vi "demo.vi"() -> ()   [LabVIEW 2016, in "mqtt.lvlib"]
uses:
  mqtt.lvlib
panel:
  in  "payload":string="Some message"
  in  "topicToPublish":string="test/device1"
  in  "topic":string="test/#"
  out "received":T1
  in  "sendSubscribe":bool
  in  "sendPublish":bool
  # "Subscribe"
  # "Subscribe"
  # "1. Connect to mqtt broker (server) by running mqtt.py\n2. Run this vi\n3. Subscribe to a topic\n4. Publish to the topic and it will be received by this vi\n5. Close panel to stop vi"
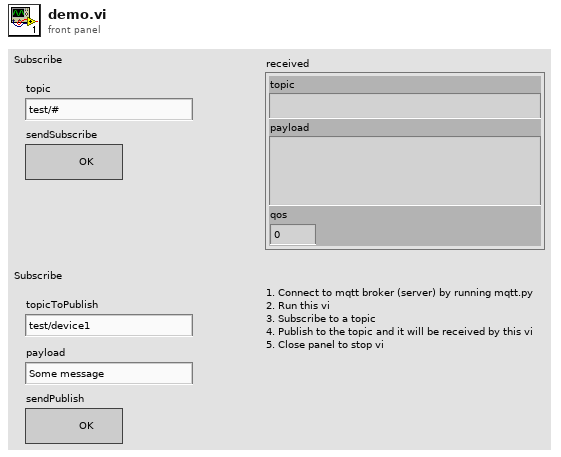
[diagram p1: front panel]
types:
  T1 = cluster{"topic":string, "payload":string, "qos":i32}
  T2 = enum16{"big-endian, network order", "native, host order", "little-endian"}
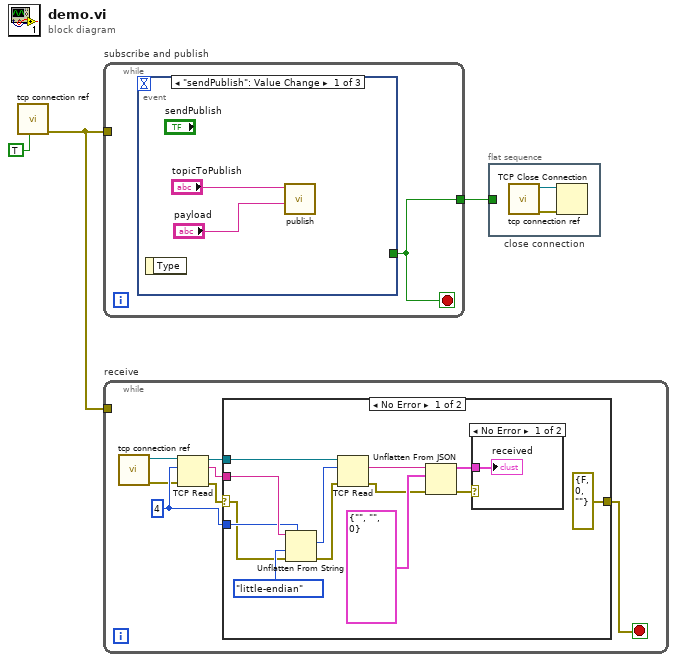
[diagram p0: block diagram]
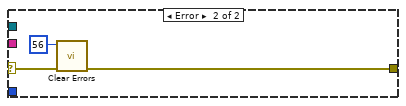
[diagram p3: hidden frame]
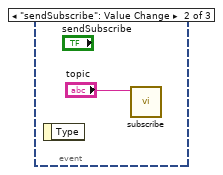
[diagram p4: hidden frame]
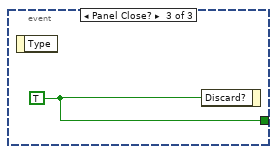
[diagram p5: hidden frame]
diagram:
  n1 = call "tcp connection ref.vi"("init"=TRUE) -> ("Error Out"=w2:errorcluster)  [unwired: 9 in, 1 out]
  n2 = while "subscribe and publish" {
    tunnel: w2 -> [_]
    tunnel: [w4] -> w1
    stop <- w4 stop-if-true
    n3 = event shown="[0] \"sendPublish\": Value Change" {
      selector: _ -> [_ _ _]
      dyn-events: _ -> [_ _ _]
      timeout: _ -> [_ _ _]
      tunnel: [_ _ w8] -> w4
      event "sendPublish": Value Change {
        n4 = event-data() -> ()  [unwired: 1 in, 1 out]
        n5 = call "publish.vi"("payload (something)"="payload", "topic (test/device1)"="topicToPublish") -> ()  [unwired: 9 in, 1 out]
      }
      event "sendSubscribe": Value Change {
        n6 = event-data() -> ()  [unwired: 1 in, 1 out]
        n7 = call "subscribe.vi"("topic (test/#)"="topic") -> ()  [unwired: 10 in, 1 out]
      }
      event Panel Close? {
        w8 = TRUE ("Discard?")
        n8 = event-data() -> ()  [unwired: 1 in, 1 out]
        n9 = event-data("Discard?"=w8) -> ()  [unwired: 1 in, 1 out]
      }
    }
  }
  n10 = while "receive" {
    tunnel: w2 -> [_]
    stop <- w9 stop-if-true
    w13 = 4 ("bytes to read")
    n11 = call "tcp connection ref.vi"() -> ("Error Out"=w11:errorcluster, "tcpRef"=w10:refnum<k5>)  [unwired: 10 in]
    n12 = TCP Read(connection ID=w10, bytes to read=w13, error in (no error)=w11) -> (connection ID out=w12:refnum<k5>, data out=w14:string, error out=w15:errorcluster)  [unwired: 2 in]
    n13 = case shown="No Error" w15 {
      selector: w15 -> [w19 w31]
      tunnel: w14 -> [w28 _]
      tunnel: w13 -> [w27 _]
      tunnel: w12 -> [w25 _]
      tunnel: [errorcluster {"status"=FALSE, "code"=0, "source"=""} ("error out") w30] -> w9
      frame No Error {
        n14 = Unflatten From String(type=w27, binary string=w28, byte order (0:big-endian, network order)=T2."little-endian", error in (no error)=w19) -> (value=w24:i32, error out=w18:errorcluster)  [unwired: 1 in, 1 out]
        n15 = TCP Read(connection ID=w25, bytes to read=w24, error in (no error)=w18) -> (data out=w23:string, error out=w17:errorcluster)  [unwired: 2 in, 1 out]
        n16 = Unflatten From JSON(JSON string=w23, type and defaults=T1 {"topic"="", "payload"="", "qos"=0}, error in (no error)=w17) -> (value=w21:T1, error out=w16:errorcluster)  [unwired: 4 in]
        n17 = case shown="No Error" w16 {
          tunnel: w21 -> [w29 _]
          frame No Error {
            "received" <- w29
          }
          frame Error {
          }
        }
      }
      frame Error {
        n18 = call <vilib>:"Clear Errors.vi"("error in (no error)"=w31, "specific error code to clear (0: all)"=56) -> ("error out"=w30:errorcluster)  [unwired: 4 in, 1 out]
      }
    }
  }
  n19 = flat-sequence "close connection" {
    tunnel: w1 -> [_]
    frame #0 {
      n20 = call "tcp connection ref.vi"() -> ("Error Out"=w34:errorcluster, "tcpRef"=w33:refnum<k5>)  [unwired: 10 in]
      n21 = TCP Close Connection(connection ID=w33, error in (no error)=w34) -> ()  [unwired: 1 in, 2 out]
    }
  }
